vi "PWM Stop.vi"(8 "error in (no error)":errorcluster, 10 "ChannelMask":u8, 11 "DevHandle":i32) -> (0 "error out":errorcluster, 3 "function return":i32)   [LabVIEW 2010, in "usb2pwm.lvlib"]
doc: "int WINAPI PWM_Stop(int DevHandle,unsigned char ChannelMask);"
uses:
  usb2pwm.lvlib
  libs/msvc_x86/USB2XXX.dll
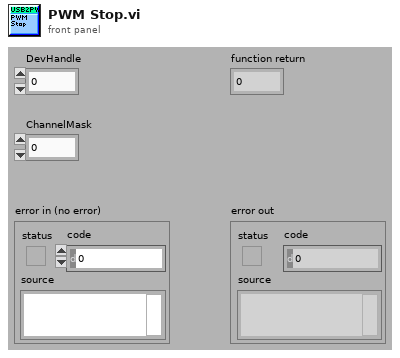
[diagram p1: front panel]
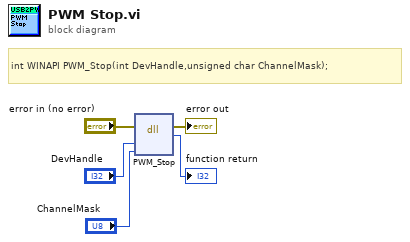
[diagram p0: block diagram]
diagram:
  # "int WINAPI PWM_Stop(int DevHandle,unsigned char ChannelMask);"
  n1 = dll-call lib="E:/OtherWork/STM32/USB2XXX_Example/sdk/libs/msvc_x86/USB2XXX.*" fn="PWM_Stop"(error in="error in (no error)", "DevHandle"="DevHandle", "ChannelMask"="ChannelMask") -> (error out=→"error out":errorcluster, →"function return":i32)  [unwired: 4 in, 1 out]
